vi "kvCanIoCtlSetTimerScale.vi"(2 "error in (no error)":errorcluster, 3 "Timestamp Clock Resolution (micro sec)":u32, 4 "Channel Handle (input only)":i32) -> (0 "error out":errorcluster, 1 "Channel Handle (ouput only)":i32)   [LabVIEW 2022 SP3]
doc: "Set the desired time-stamp clock resolution in microseconds. Note that the accuracy of the clock isn't affected. The default value is 1000 microseconds, i.e. one millisecond."
uses:
  canlib32.dll
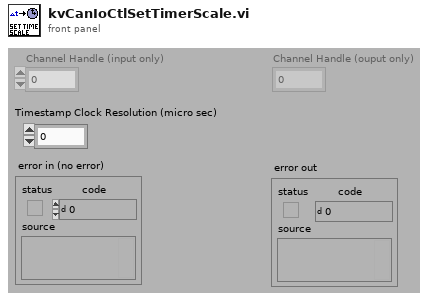
[diagram p1: front panel]
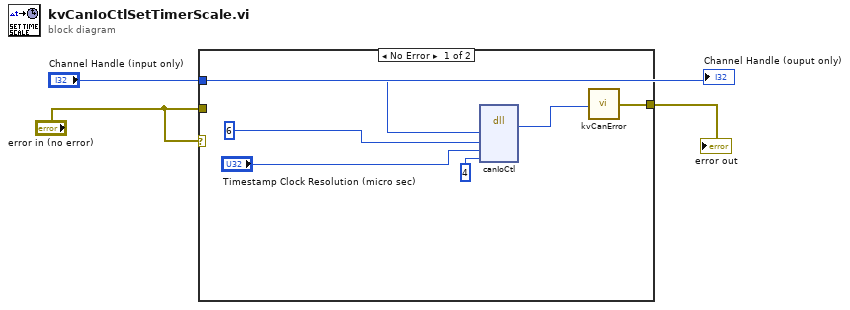
[diagram p0: block diagram]
diagram:
  n1 = case shown="No Error" "error in (no error)" {
    tunnel: [w9 w10] -> w3
    tunnel: "error in (no error)" -> [_ w10]
    tunnel: "Channel Handle (input only)" -> [w7 _]
    frame No Error {
      n2 = dll-call lib="canlib32.dll" fn="canIoCtl" label="Call canIoCtl"("handle"=w7, "func"=6, "buf"="Timestamp Clock Resolution (micro sec)", "buflen"=4) -> (w8:i32)  [unwired: 7 in, 2 out]
      n3 = call "kvCanError.vi"("error code"=w8) -> ("error out"=w9:errorcluster)
    }
    frame Error {
    }
  }
  "error out" <- w3
  "Channel Handle (ouput only)" <- "Channel Handle (input only)"
